vi "SV Match Unit.vi"(8 "error in (no error)":errorcluster, 10 "Units to Match":string[](array[string]), 11 "scaled signal [EU]":waveform(dbl)={"t0"=timestamp(0 s since 1904-01-01), "dt"=0.0, "Y"=[]}) -> (0 "error out":errorcluster, 1 "unit label":string, 2 "Found?":bool, 3 "dup scaled signal [EU]":waveform(dbl))   [LabVIEW 2017]
uses:
  <vilib>/addons/_NISVFA/_Shared subVIs/Controls/NI Channel Properties.ctl
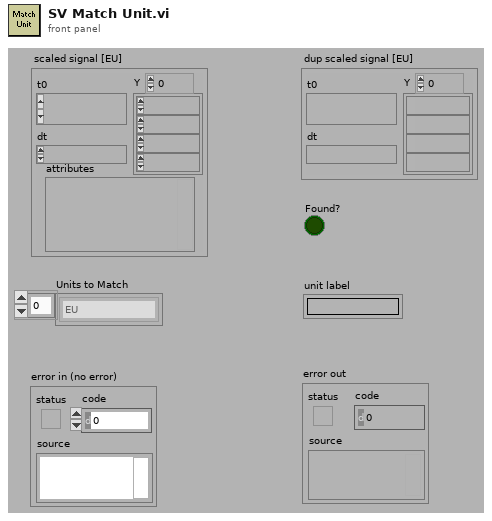
[diagram p1: front panel]
types:
  T1 = typedef "NI Channel Properties.ctl" = u16
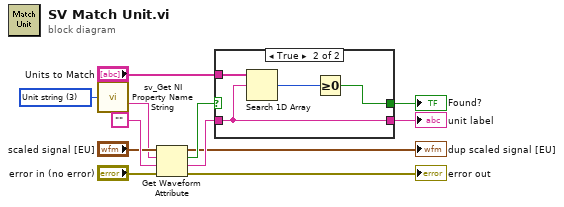
[diagram p0: block diagram]
diagram:
  w2 = T1 3 items=["Channel name", "Channel description", "Axis label", "Unit string", "Waveform X-axis label", "Waveform X-axis unit string", "x0", "dx", "Number of samples", "X channel", "Filter settled", "dB reference", "Window", "Window parameter", "Window size", "FFT size", "Peak units", "Spectrum type", "Magnitude scale", "Spectral density", "Sensor sensitivity (mV/EU)", "X-axis dimension", "LabVIEW datatype", "Function type", "Function subtype", "X values", "Independent channel", "Column index", "Collection name", "Collection ID", "X Columns", "Phase unwrapped"] ("property")
  n1 = call <vilib>:"sv_Get NI Property Name String.vi"("property"=w2) -> ("WDT attribute name"=w1:string)  [unwired: 13 in, 1 out]
  n2 = Get Waveform Attribute(4:"error in (no error)", 5:"" ("Empty String Constant"), 6:w1, 7:"scaled signal [EU]") -> (0:→"error out":errorcluster, 1:w8:string, 2:w9:bool, 3:→"dup scaled signal [EU]":waveform(dbl))
  n3 = case shown="True" w9 {
    selector: w9 -> [w13 _]
    tunnel: w8 -> [w14 w17]
    tunnel: "Units to Match" -> [_ w18]
    tunnel: [w13 w15] -> w6
    tunnel: [w14 w17] -> w5
    frame False {
    }
    frame True {
      n4 = Search 1D Array(1D array=w18, element=w17) -> (index of element=w16:i32)  [unwired: 1 in]
      n5 = Greater Or Equal To 0?(x=w16) -> (x >= 0?=w15:bool)
    }
  }
  "unit label" <- w5
  "Found?" <- w6
